vi "Jog a Motor.vi"(0 "Motions in":refnum<class "Motions.lvclass">, 5 "Index":i32, 7 "Dir":string(combo)="+", 9 "Amplitude":u16, 11 "error in (no error)":errorcluster) -> (4 "Motions out":refnum<class "Motions.lvclass">, 15 "error out":errorcluster)   [LabVIEW 2016, in "Hardware.lvlib" / "Motions.lvlib" / "Motions.lvclass"]
uses:
  <userlib>/Common Components/Hardware/Abstract System/Motions/Motions/Motions.lvclass
  <userlib>/Common Components/Hardware/Abstract System/Motions/Motions/Motions.lvclass/Motions.ctl
  <userlib>/Common Components/Hardware/Motor/Motor/Motor.lvclass/Motor.ctl
  <userlib>/Common Components/Hardware/Motor/Motor/Accessor/Read soft limit max.vi
  <userlib>/Common Components/Hardware/Motor/Motor/Accessor/Read soft limit min.vi
  <userlib>/Common Components/Hardware/Motor/Motor/Accessor/Read motor pulses per revolution.vi
  <userlib>/Common Components/Hardware/Motor/Motor/Accessor/Read Achievable Steps per Rev.vi
  <userlib>/Common Components/Hardware/Motor/Motor/Motor.lvclass
panel:
  # "a seekbar with range 1-100"
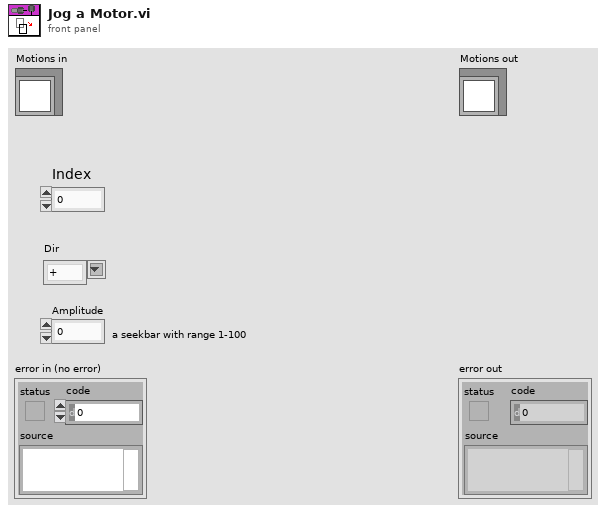
[diagram p1: front panel]
types:
  T1 = typedef "Hardware.lvlib/Motions.lvlib/Motions.lvclass/Motor States.ctl" = cluster{"Connected":bool, "Enabled":bool, "Moving Status":bool, "Soft Moving Status":bool, "Current Pos":dbl, "Target Pos":dbl, "Moving Dir (-1, 0, 1)":i32, "Error Status":bool, "Hard Limit+":bool, "Hard Limit-":bool, "Soft Limit+":bool, "Soft Limit-":bool, "History Dst Stack":refnum<queue>, "Motion Status":bool, "Motion TriggerAction Obj":refnum<class "TriggerAction Q.lvclass">, "Jogging":bool}
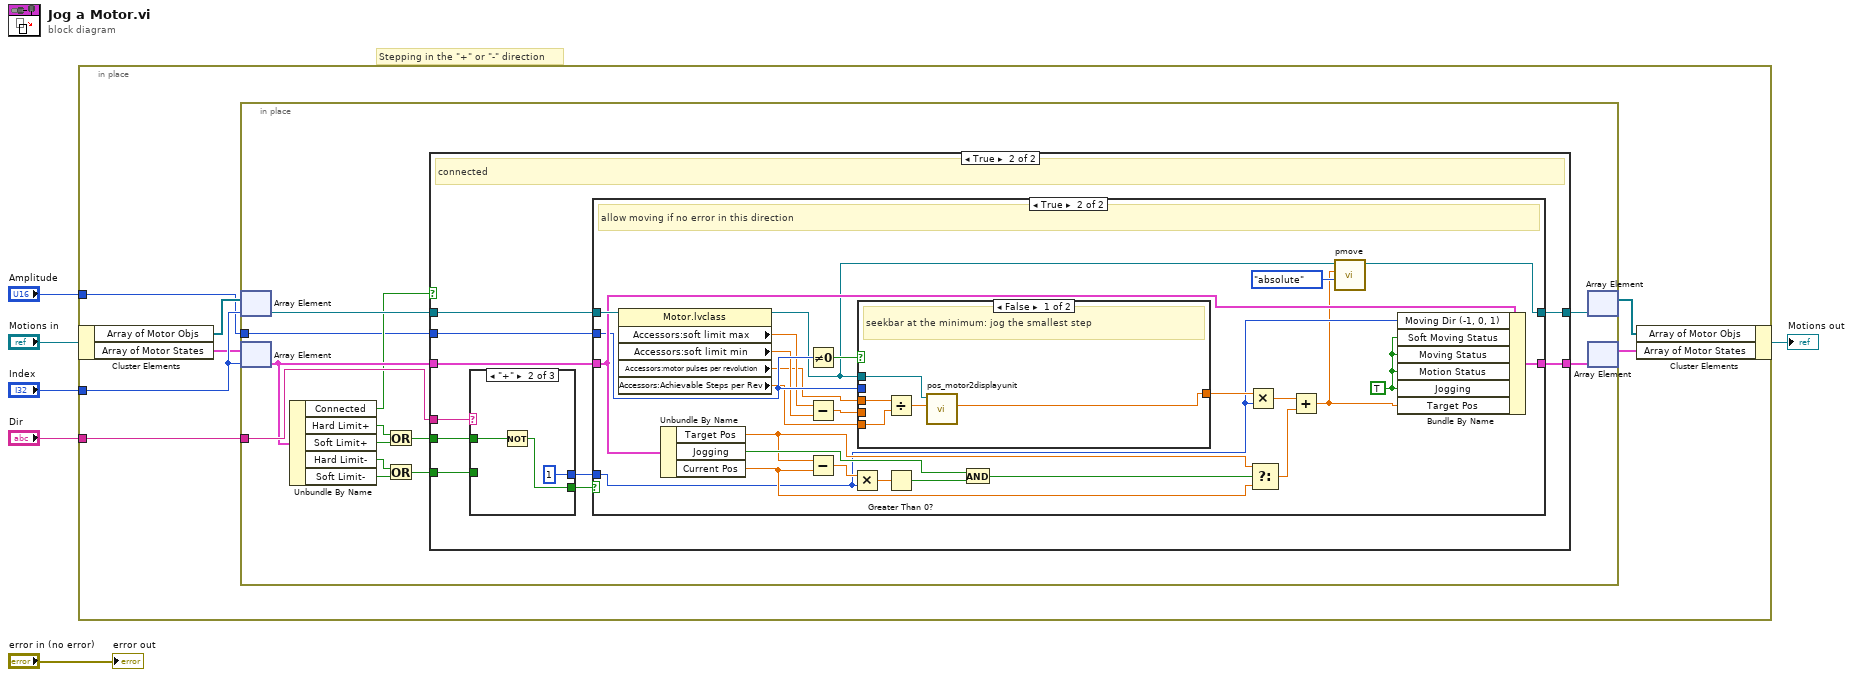
[diagram p0: block diagram]
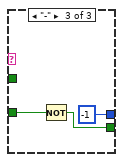
[diagram p4: hidden frame]
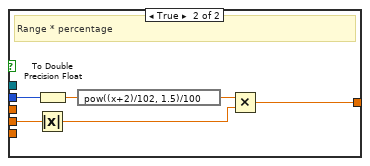
[diagram p6: hidden frame]
diagram:
  # "Stepping in the \"+\" or \"-\" direction"
  n1 = in-place {
    in-place-border: "Index" -> [w10]
    in-place-border: "Dir" -> [w11]
    in-place-border: "Amplitude" -> [w7]
    n2 = in-place-cluster #1("Motions in") -> ("Array of Motor Objs"=w13:refnum<class "Motor.lvclass">[], "Array of Motor States"=w9:T1[])
    n3 = in-place {
      in-place-border: w11 -> [w25]
      in-place-border: w7 -> [w14]
      n4 = in-place-array #2(w13, w10) -> (w26:refnum<class "Motor.lvclass">)
      n5 = in-place-array #3(w9, w10) -> (w24:T1)
      n6 = Unbundle By Name(w24) -> ("Connected"=w22:bool, "Hard Limit+"=w20:bool, "Soft Limit+"=w19:bool, "Hard Limit-"=w18:bool, "Soft Limit-"=w17:bool)
      n7 = Or(x=w20, y=w19) -> (x .or. y?=w16:bool)
      n8 = Or(x=w18, y=w17) -> (x .or. y?=w15:bool)
      n9 = case shown="True" w22 {
        tunnel: w26 -> [w27 w36]
        tunnel: w25 -> [_ w31]
        tunnel: w24 -> [w28 w38]
        tunnel: [w28 w37] -> w23
        tunnel: [w27 w35] -> w21
        tunnel: w16 -> [_ w33]
        tunnel: w15 -> [_ w32]
        tunnel: w14 -> [_ w29]
        frame False {
        }
        frame True {
          # "connected"
          n10 = case shown="\"+\"" w31 {
            tunnel: [_ w40 w43] -> w34
            tunnel: w33 -> [_ w41 _]
            tunnel: w32 -> [_ _ w44]
            tunnel: [_ 1 -1] -> w30
            frame Default {
            }
            frame "+" {
              n11 = Not(x=w41) -> (.not. x?=w40:bool)
            }
            frame "-" {
              n12 = Not(x=w44) -> (.not. x?=w43:bool)
            }
          }
          n13 = case shown="True" w34 {
            tunnel: w30 -> [_ w52]
            tunnel: w38 -> [w45 w68]
            tunnel: [w45 w72] -> w37
            tunnel: w36 -> [w46 w70]
            tunnel: [w46 w71] -> w35
            tunnel: w29 -> [_ w65]
            frame False {
            }
            frame True {
              w47 = TRUE ("Soft Moving Status")
              # "allow moving if no error in this direction"
              n14 = property class="Motor.lvclass"(reference=w70) -> (reference out=w58:refnum<class "Motor.lvclass">, "Accessors:soft limit max"=w64:dbl, "Accessors:soft limit min"=w63:dbl, "Accessors:motor pulses per revolution"=w60:dbl, "Accessors:Achievable Steps per Rev"=w59:dbl)  [unwired: 1 in, 1 out]
              n15 = Unbundle By Name(w68) -> ("Target Pos"=w55:dbl, "Jogging"=w67:bool, "Current Pos"=w54:dbl)
              n16 = Not Equal To 0?(x=w65) -> (x != 0?=w66:bool)
              n17 = Subtract(x=w64, y=w63) -> (x-y=w62:dbl)
              n18 = Subtract(x=w55, y=w54) -> (x-y=w53:dbl)
              n19 = Multiply(x=w53, y=w52) -> (x*y=w51:dbl)
              n20 = case shown="False" w66 {
                tunnel: w65 -> [_ w83]
                tunnel: w62 -> [_ w79]
                tunnel: [w73 w81] -> w61
                tunnel: w60 -> [w77 _]
                tunnel: w59 -> [w76 _]
                tunnel: w58 -> [w75 _]
                frame False {
                  # "seekbar at the minimum: jog the smallest step"
                  n21 = Divide(x=w77, y=w76) -> (x/y=w74:dbl)
                  n22 = call <userlib>:"pos_motor2displayunit.vi"("pos in motor (pulses)"=w74, "Motor in"=w75) -> ("pos in display unit"=w73:dbl)  [unwired: 7 in, 2 out]
                }
                frame True {
                  # "Range * percentage"
                  n23 = Absolute Value(x=w79) -> (abs(x)=w78:dbl)
                  n24 = To Double Precision Float(number=w83) -> (double precision float=w82:dbl)
                  n25 = expression code="pow((x+2)/102, 1.5)/100"(w82) -> (w80:dbl)
                  n26 = Multiply(x=w80, y=w78) -> (x*y=w81:dbl)
                }
              }
              n27 = Greater Than 0?(x=w51) -> (x > 0?=w49:bool)
              n28 = And(x=w67, y=w49) -> (x .and. y?=w50:bool)
              n29 = Multiply(x=w61, y=w52) -> (x*y=w56:dbl)
              n30 = Select(t=w55, s=w50, f=w54) -> (s? t:f=w57:dbl)
              n31 = Add(x=w56, y=w57) -> (x+y=w48:dbl)
              n32 = call <userlib>:"pmove.vi"("mode (0: rel; 1: abs)"=enum16{"relative", "absolute"}."absolute", "distance in display unit"=w48, "Motor in"=w58) -> ("Motor out"=w71:refnum<class "Motor.lvclass">)  [unwired: 7 in, 1 out]
              n33 = Bundle By Name(cluster=w68, "Moving Dir (-1, 0, 1)"=w52, "Soft Moving Status"=w47, "Moving Status"=w47, "Motion Status"=w47, "Jogging"=w47, "Target Pos"=w48) -> (w72:T1)
            }
          }
        }
      }
      n34 = in-place-array #2(w21) -> (w12:refnum<class "Motor.lvclass">[])  [unwired: 1 out]
      n35 = in-place-array #3(w23) -> (w8:T1[])  [unwired: 1 out]
    }
    n36 = in-place-cluster #1("Array of Motor Objs"=w12, "Array of Motor States"=w8) -> (→"Motions out":refnum<class "Motions.lvclass">)
  }
  "error out" <- "error in (no error)"
